vi "QR_code_Check.vi"(5 "Columns":string[](array[string]), 6 "format string":string, 7 "error in (no error)":errorcluster, 8 "replace %s":string, 9 "table":string, 10 "Refnum in":T1) -> (0 "error out":errorcluster, 1 "data":string[][](array[string]), 2 "FALSE healty":bool, 3 "Refnum out":T1, 4 "TRUE Duplication on Station 2":bool)   [LabVIEW 2017]
uses:
  <vilib>/addons/database/Connection.llb/Conn ObjectReference.ctl
  <vilib>/addons/database/NI_Database_API.lvlib
panel:
  out "TRUE no barcode Done on station 1":bool
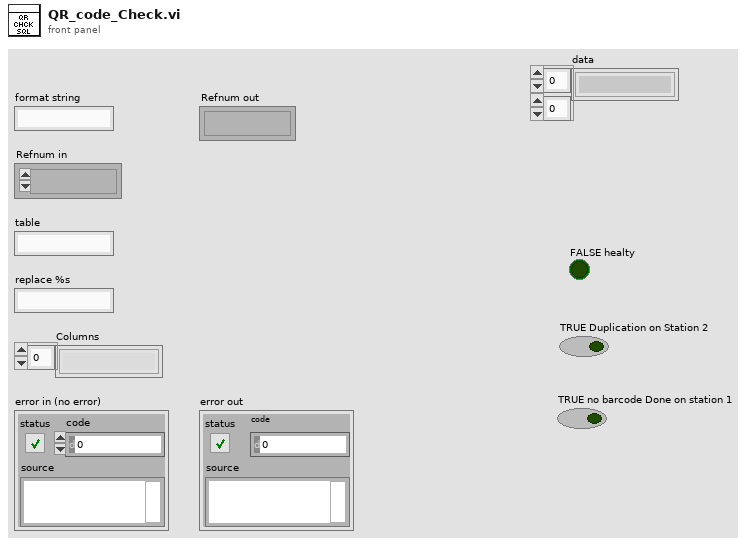
[diagram p1: front panel]
types:
  T1 = typedef "NI_Database_API.lvlib/Conn ObjectReference.ctl" = refnum<k1>
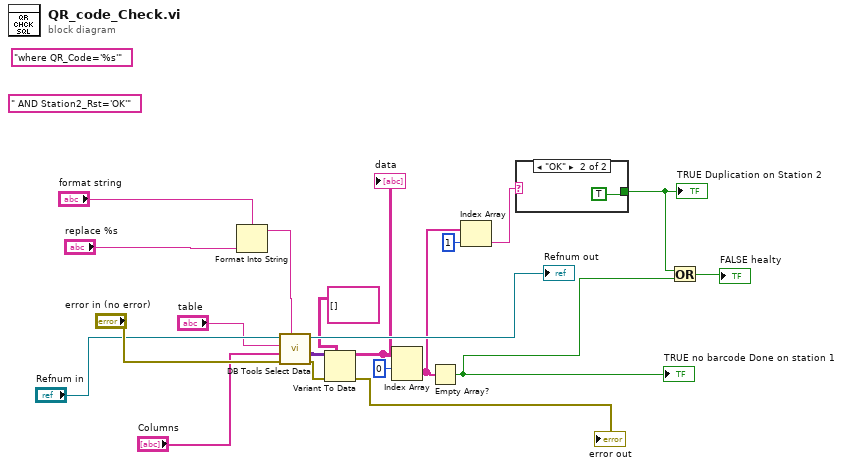
[diagram p0: block diagram]
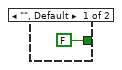
[diagram p2: hidden frame]
diagram:
  (unwired) "where QR_Code='%s'" ("format string")
  (unwired) " AND Station2_Rst='OK'" ("replace %s")
  n1 = Format Into String(format string="format string", "replace %s") -> (resulting string=w7:string)  [unwired: 2 in, 1 out]
  n2 = call <vilib>:"DB Tools Select Data.vi"("condition"=w7, "error in (no error)"="error in (no error)", "columns"="Columns", "table"="table", "connection reference"="Refnum in") -> ("error out"=w8:errorcluster, "data"=w10:variant[][], "connection reference out"=→"Refnum out":T1)  [unwired: 1 in]
  n3 = Variant To Data(error in=w8, type=string[][] [], Variant=w10) -> (data=w9:string[][], error out=→"error out":errorcluster)
  "data" <- w9
  n4 = Index Array(array=w9, index (row)=0) -> (element=w5:string[])  [unwired: 1 in]
  n5 = Empty Array?(array=w5) -> (empty?=w2:bool)
  "TRUE no barcode Done on station 1" <- w2
  n6 = Index Array(array=w5, index=1 ("index (row)")) -> (element=w4:string)
  n7 = case shown="\"OK\"" w4 {
    tunnel: [FALSE TRUE] -> w1
    frame "", Default {
    }
    frame "OK" {
    }
  }
  "TRUE Duplication on Station 2" <- w1
  n8 = Or(x=w1, y=w2) -> (x .or. y?=→"FALSE healty":bool)
